vi "Set Motor Modes.vi"(0 "Drive/Climb State":T4, 2 "Robot Commands":T1, 7 "Ball Gatherer State":T5, 11 "Shooter State":T3) -> (4 "Drive/Climb State Out":T4, 8 "Ball Gatherer State Out":T5, 15 "Shooter State Out":T3)   [LabVIEW 2015]
uses:
  Load SS/Ball Gatherer State.ctl
  Drive SS/Drive Subsystem State.ctl
  Shoot SS/Shooter Control.ctl
  Robot Commands 2016.ctl
  Load SS/Roller State.ctl
  <vilib>/Rock Robotics/WPI/CAN/TalonSRX/WPI_CANTalonSRX_APIControlMode.ctl
  Global Variables/Temp Variables.vi
  Global Variables/Calibrations.vi
  Global Variables/refnum names.vi
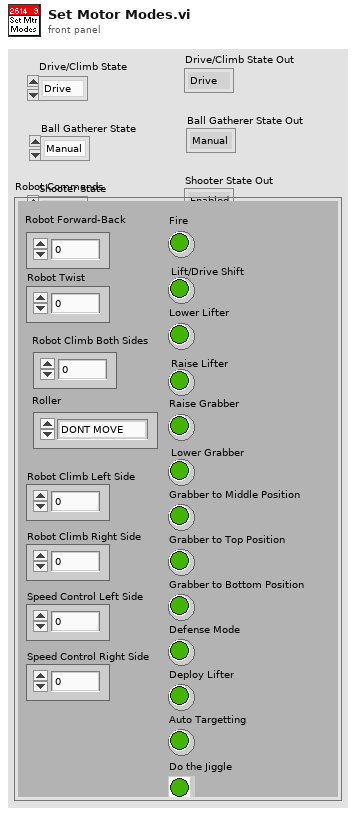
[diagram p1: front panel]
types:
  T1 = typedef "Robot Commands 2016.ctl" = cluster{"Robot Forward-Back":dbl, "Robot Twist":dbl, "Fire":bool, "Lift/Drive Shift":bool, "Raise Lifter":bool, "Raise Grabber":bool, "Lower Grabber":bool, "Roller":T2, "Robot Climb Both Sides":dbl, "Grabber to Middle Position":bool, "Grabber to Top Position":bool, "Grabber to Bottom Position":bool, "Robot Climb Left Side":dbl, "Robot Climb Right Side":dbl, "Speed Control Left Side":dbl, "Speed Control Right Side":dbl, "Lower Lifter":bool, "Defense Mode":bool, "Deploy Lifter":bool, "Auto Targetting":bool, "Do the Jiggle":bool}
  T2 = typedef "Roller State.ctl" = enum16{"DONT MOVE", "Intake", "Outtake"}
  T3 = typedef "Shooter Control.ctl" = enum16{"Enabled", "Disabled"}
  T4 = typedef "Drive Subsystem State.ctl" = enum16{"Drive", "Climb", "Auto Target"}
  T5 = typedef "Ball Gatherer State.ctl" = enum16{"Manual", "Positional"}
  T6 = typedef "WPI_MotorControlDeviceRef.ctl" = cluster{"DeviceStatus":errorcluster, "Type":T7, "PWM":cluster{"PWM Channel":T8, "DeadBand":T9}, "CAN":cluster{"Device Number":u8, "Control Mode":T10, "Semaphore":T11, "Max Vout":dbl, "TalonSRX Control Mode":T12}, "Invert":bool}
  T7 = typedef "WPI_MotorControlType.ctl" = enum16{"PWM", "CAN", "CANTalonSRX"}
  T8 = typedef "FPGA_DIOPWMChannel.ctl" = enum8{"PWM 0", "PWM 1", "PWM 2", "PWM 3", "PWM 4", "PWM 5", "PWM 6", "PWM 7", "PWM 8", "PWM 9", "PWM MXP 0", "PWM MXP 1", "PWM MXP 2", "PWM MXP 3", "PWM MXP 4", "PWM MXP 5", "PWM MXP 6", "PWM MXP 7", "PWM MXP 8", "PWM MXP 9", "Invalid"}
  T9 = typedef "WPI_PWMDeadband.ctl" = cluster{"Name":string, "maxPositivePwm":i32, "minPositivePwm":i32, "centerPwm":i32, "maxNegativePwm":i32, "minNegativePwm":i32, "angularRange":u16}
  T10 = typedef "WPI_CANJaguar_ControlMode.ctl" = enum8{"Percent VBus", "Current", "Speed", "Position", "Voltage"}
  T11 = typedef "Semaphore RefNum" = refnum<k1>
  T12 = typedef "WPI_CANTalonSRX_APIControlMode.ctl" = enum8{"Percent VBus", "Speed", "Position", "Slave", "Unchanged / Invalid", "Voltage Compensation", "Current", "Motion Profile"}
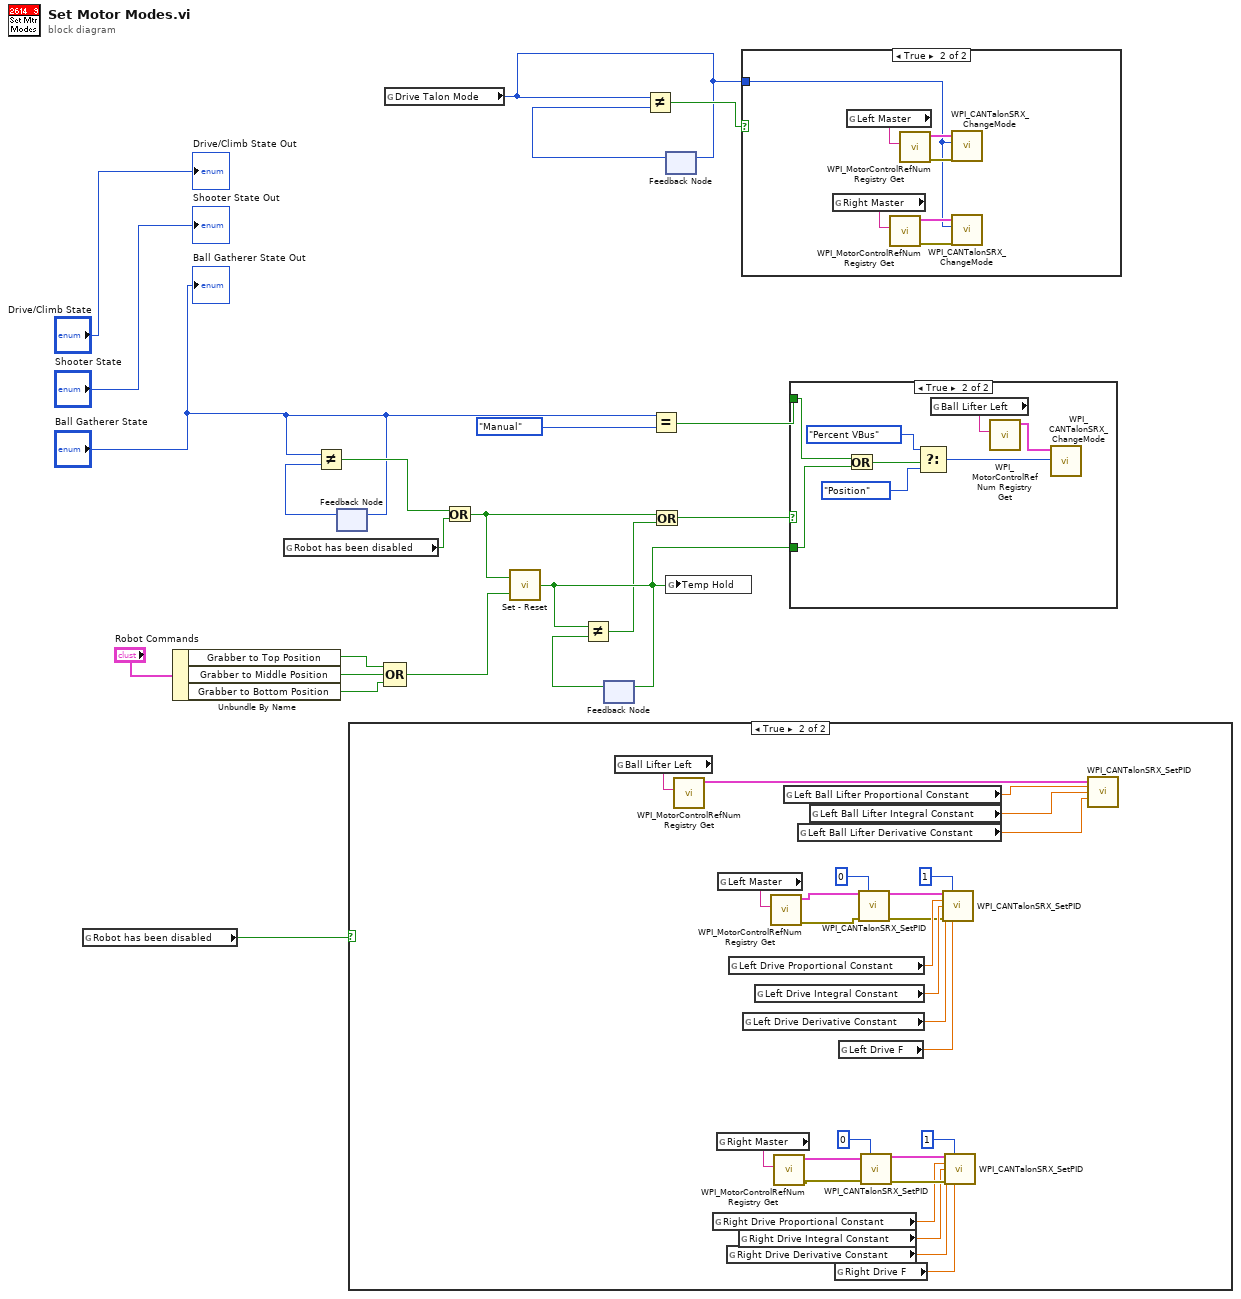
[diagram p0: block diagram]
diagram:
  n1 = global read "Temp Variables.vi" "Robot has been disabled"() -> (w7:bool)
  n2 = Unbundle By Name("Robot Commands") -> ("Grabber to Top Position"=w13:bool, "Grabber to Middle Position"=w12:bool, "Grabber to Bottom Position"=w11:bool)
  n3 = global read "Temp Variables.vi" "Robot has been disabled"() -> (w15:bool)
  n4 = feedback #1() -> (w17:T5)  [unwired: 1 in]
  n5 = Not Equal?(x="Ball Gatherer State", y=w17) -> (x != y?=w16:bool)
  n6 = feedback-in #1("Ball Gatherer State") -> ()
  n7 = case shown="True" w7 {
    frame False {
    }
    frame True {
      n8 = global read "refnum names.vi" "Ball Lifter Left"() -> (w46:string)
      n9 = call <vilib>:"WPI_MotorControlRefNum Registry Get.vi"("refnum name"=w46) -> ("MotorControlDevRef"=w45:T6)  [unwired: 9 in, 1 out]
      n10 = global read "Calibrations.vi" "Right Drive Proportional Constant"() -> (w39:dbl)
      n11 = global read "refnum names.vi" "Right Master"() -> (w26:string)
      n12 = global read "refnum names.vi" "Left Master"() -> (w44:string)
      n13 = global read "Calibrations.vi" "Right Drive Derivative Constant"() -> (w41:dbl)
      n14 = global read "Calibrations.vi" "Left Drive Proportional Constant"() -> (w34:dbl)
      n15 = global read "Calibrations.vi" "Right Drive Integral Constant"() -> (w40:dbl)
      n16 = global read "Calibrations.vi" "Left Drive Derivative Constant"() -> (w36:dbl)
      n17 = global read "Calibrations.vi" "Left Drive Integral Constant"() -> (w35:dbl)
      n18 = call <vilib>:"WPI_MotorControlRefNum Registry Get.vi"("refnum name"=w44) -> ("error out"=w24:errorcluster, "MotorControlDevRef"=w25:T6)  [unwired: 9 in]
      n19 = call <vilib>:"WPI_MotorControlRefNum Registry Get.vi"("refnum name"=w26) -> ("error out"=w28:errorcluster, "MotorControlDevRef"=w27:T6)  [unwired: 9 in]
      n20 = global read "Calibrations.vi" "Left Ball Lifter Proportional Constant"() -> (w49:dbl)
      n21 = global read "Calibrations.vi" "Left Ball Lifter Derivative Constant"() -> (w47:dbl)
      n22 = global read "Calibrations.vi" "Left Ball Lifter Integral Constant"() -> (w48:dbl)
      n23 = global read "Calibrations.vi" "Right Drive F"() -> (w42:dbl)
      n24 = global read "Calibrations.vi" "Left Drive F"() -> (w37:dbl)
      n25 = call <vilib>:"WPI_CANTalonSRX_SetPID.vi"("CAN Talon SRX Ref"=w25, "Parameter Slot"=u8 0, "error in (no error)"=w24) -> ("CAN Talon SRX Ref"=w33:T6, "error out"=w23:errorcluster)  [unwired: 11 in]
      n26 = call <vilib>:"WPI_CANTalonSRX_SetPID.vi"("CAN Talon SRX Ref"=w27, "Parameter Slot"=u8 0, "error in (no error)"=w28) -> ("CAN Talon SRX Ref"=w31:T6, "error out"=w43:errorcluster)  [unwired: 11 in]
      n27 = call <vilib>:"WPI_CANTalonSRX_SetPID.vi"("CAN Talon SRX Ref"=w33, "Parameter Slot"=u8 1, "P"=w34, "I"=w35, "D"=w36, "error in (no error)"=w23, "F"=w37) -> ()  [unwired: 7 in, 2 out]
      n28 = call <vilib>:"WPI_CANTalonSRX_SetPID.vi"("CAN Talon SRX Ref"=w31, "Parameter Slot"=u8 1, "P"=w39, "I"=w40, "D"=w41, "error in (no error)"=w43, "F"=w42) -> ()  [unwired: 7 in, 2 out]
      n29 = call <vilib>:"WPI_CANTalonSRX_SetPID.vi"("CAN Talon SRX Ref"=w45, "P"=w49, "I"=w48, "D"=w47) -> ()  [unwired: 10 in, 2 out]
    }
  }
  n30 = Compound Arithmetic op=OR(w13, w12, w11) -> (w10:bool)
  n31 = global read "Temp Variables.vi" "Drive Talon Mode"() -> (w18:T12)
  n32 = Or(x=w16, y=w15) -> (x .or. y?=w3:bool)
  n33 = call "Set - Reset.vi"("Reset"=w10, "Set"=w3) -> ("Output"=w4:bool)
  n34 = feedback #2() -> (w5:bool)  [unwired: 1 in]
  n35 = Not Equal?(x=w4, y=w5) -> (x != y?=w1:bool)
  n36 = feedback-in #2(w4) -> ()
  n37 = Equal?(x="Ball Gatherer State", y=Ball_Gatherer_State."Manual") -> (x = y?=w8:bool)
  n38 = Or(x=w3, y=w1) -> (x .or. y?=w2:bool)
  n39 = feedback-in #3(w18) -> ()
  n40 = feedback #3() -> (w20:T12)  [unwired: 1 in]
  n41 = Not Equal?(x=w18, y=w20) -> (x != y?=w19:bool)
  n42 = global write "Temp Variables.vi" "Temp Hold"(w4) -> ()
  n43 = case shown="True" w19 {
    tunnel: w18 -> [_ w50]
    frame False {
    }
    frame True {
      n44 = global read "refnum names.vi" "Right Master"() -> (w53:string)
      n45 = global read "refnum names.vi" "Left Master"() -> (w56:string)
      n46 = call <vilib>:"WPI_MotorControlRefNum Registry Get.vi"("refnum name"=w53) -> ("error out"=w52:errorcluster, "MotorControlDevRef"=w51:T6)  [unwired: 9 in]
      n47 = call <vilib>:"WPI_MotorControlRefNum Registry Get.vi"("refnum name"=w56) -> ("error out"=w55:errorcluster, "MotorControlDevRef"=w54:T6)  [unwired: 9 in]
      n48 = call <vilib>:"WPI_CANTalonSRX_ChangeMode.vi"("error in (no error)"=w55, "Control Mode"=w50, "CAN Talon SRX Ref"=w54) -> ()  [unwired: 7 in, 2 out]
      n49 = call <vilib>:"WPI_CANTalonSRX_ChangeMode.vi"("error in (no error)"=w52, "Control Mode"=w50, "CAN Talon SRX Ref"=w51) -> ()  [unwired: 7 in, 2 out]
    }
  }
  n50 = case shown="True" w2 {
    tunnel: w8 -> [_ w61]
    tunnel: w4 -> [_ w60]
    frame False {
    }
    frame True {
      n51 = Or(x=w61, y=w60) -> (x .or. y?=w62:bool)
      n52 = Select(t=WPI_CANTalonSRX_APIControlMode."Percent VBus" ("Drive Talon Mode"), s=w62, f=WPI_CANTalonSRX_APIControlMode."Position" ("Drive Talon Mode")) -> (s? t:f=w63:T12)
      n53 = global read "refnum names.vi" "Ball Lifter Left"() -> (w58:string)
      n54 = call <vilib>:"WPI_MotorControlRefNum Registry Get.vi"("refnum name"=w58) -> ("MotorControlDevRef"=w57:T6)  [unwired: 9 in, 1 out]
      n55 = call <vilib>:"WPI_CANTalonSRX_ChangeMode.vi"("Control Mode"=w63, "CAN Talon SRX Ref"=w57) -> ()  [unwired: 8 in, 2 out]
    }
  }
  "Ball Gatherer State Out" <- "Ball Gatherer State"
  "Drive/Climb State Out" <- "Drive/Climb State"
  "Shooter State Out" <- "Shooter State"
